vi "send_recieve.vi"(6 "wait ms (default 50)":u32=50, 7 "error in (no error)":errorcluster, 9 "write buffer":string, 10 "VISA resource name":refnum<visa-resource-name>) -> (0 "error out":errorcluster, 2 "read buffer":string, 3 "VISA resource name out":refnum<visa-resource-name>)   [LabVIEW 2018, in "VISA Common.lvlib"]
uses:
  VISA Common/VISA Common.lvlib
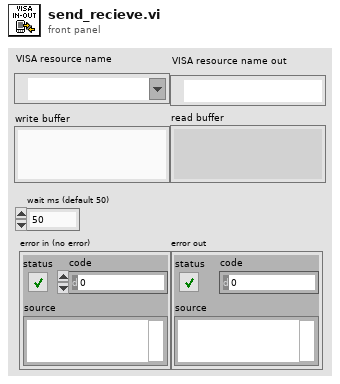
[diagram p1: front panel]
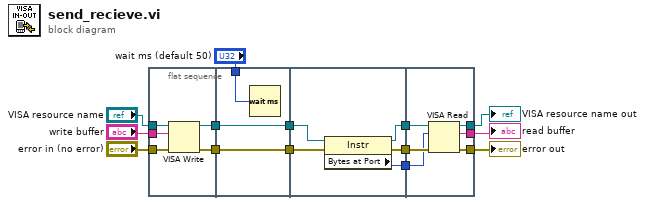
[diagram p0: block diagram]
diagram:
  n1 = flat-sequence {
    tunnel: [w19] -> w14
    tunnel: [w18] -> w13
    tunnel: "VISA resource name" -> [w17]
    tunnel: "write buffer" -> [w16]
    tunnel: "error in (no error)" -> [w15]
    tunnel: [w22] -> w12
    tunnel: w14 -> [w22]
    tunnel: [w21] -> w11
    tunnel: w13 -> [w21]
    tunnel: "wait ms (default 50)" -> [w20]
    tunnel: w12 -> [w27]
    tunnel: [w25] -> w10
    tunnel: [w26] -> w9
    tunnel: [w24] -> w8
    tunnel: w11 -> [w23]
    tunnel: [w30] -> w5
    tunnel: [w31] -> w6
    tunnel: w10 -> [w33]
    tunnel: w9 -> [w32]
    tunnel: w8 -> [w29]
    tunnel: [w28] -> w7
    frame #0 {
      n2 = VISA Write(VISA resource name=w17, write buffer=w16, error in (no error)=w15) -> (VISA resource name out=w18:refnum<visa-resource-name>, error out=w19:errorcluster)  [unwired: 1 out]
    }
    frame #1 {
      n3 = Wait (ms)(milliseconds to wait=w20) -> ()  [unwired: 1 out]
    }
    frame #2 {
      n4 = property class="Instr"(reference=w23, error in=w27) -> (reference out=w26:refnum<visa-resource-name>, error out=w25:errorcluster, "Bytes at Port"=w24:u32)
    }
    frame #3 {
      n5 = VISA Read(VISA resource name=w32, byte count=w29, error in (no error)=w33) -> (VISA resource name out=w30:refnum<visa-resource-name>, read buffer=w28:string, error out=w31:errorcluster)  [unwired: 1 out]
    }
  }
  "read buffer" <- w7
  "error out" <- w6
  "VISA resource name out" <- w5
